vi "Actor Core.vi"(8 "error in":errorcluster, 11 "State Actor in":refnum<class "State Actor.lvclass">) -> (0 "error out":errorcluster, 3 "Actor out":refnum<class "Actor.lvclass">)   [LabVIEW 2024, in "State Actor.lvlib" / "State Actor.lvclass"]
doc: "<p>(<strong>Filename</strong>: <span class=\"dnl\">Actor Framework.lvlib:Actor.lvclass:Actor Core.vi</span>)</p>\n<p>Receives messages to the actor, reacts to them, and initiates any error handling that may shut the actor down.</p>\n<p>Descendant classes may override this VI to append parallel tasks for the actor to complete while it handles messages. Overrides use the <a href=\"nihelplauncher://docs/csh?context=lvcore_glang_udclass\">Call Parent Class Method</a> node.</p>"
uses:
  State Actor.lvclass
  State Actor.lvclass/State Actor.ctl
  <vilib>/ActorFramework/Actor/Actor.lvclass
  C:/Program Files (x86)/National Instruments/LabVIEW 2024/vi.lib/ActorFramework/Actor/Actor.lvclass
  C:/Users/uspoaotto/Downloads/State Actor/State Actor/State Actor.lvclass
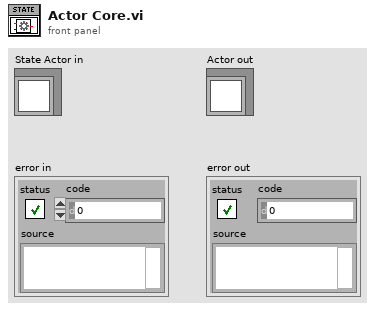
[diagram p1: front panel]
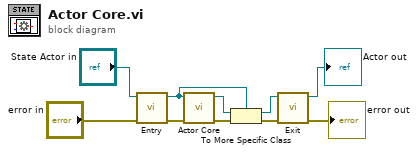
[diagram p0: block diagram]
diagram:
  n1 = call-dynamic "Entry.vi"("error in (no error)"="error in", "State Actor in"="State Actor in") -> ("error out"=w8:errorcluster, "State Actor out"=w6:refnum<class "State Actor.lvclass">)  [unwired: 8 in]
  n2 = call-parent "Actor Core.vi"("error in"=w8, "Actor in"=w6) -> ("error out"=w5:errorcluster, "Actor out"=w7:refnum<class "Actor.lvclass">)  [unwired: 8 in]
  n3 = To More Specific Class(target class=w6, reference=w7, error in=w5) -> (specific class reference=w3:refnum<class "State Actor.lvclass">, error out=w4:errorcluster)
  n4 = call-dynamic "Exit.vi"("error in (no error)"=w4, "State Actor in"=w3) -> ("error out"=→"error out":errorcluster, "State Actor out"=→"Actor out":refnum<class "State Actor.lvclass">)  [unwired: 8 in]
